vi "VNARP PARABOLA FIT.vi"(0 "Freq Table IN":dbl[](array[numeric]), 1 "Fit length":i32=500, 2 "Y IN":dbl[](array[numeric]) caption="Y") -> (3 "Best Polynomial Fit":dbl[](array[numeric]) caption="Meilleur ajustement polynomial", 4 "Parabol max position":dbl, 5 "élément":dbl, 6 "sous-tableau":dbl[](array[numeric]))   [LabVIEW 2021]
uses:
  <vilib>/Analysis/6fits.llb/General Linear Fit Algorithm.ctl
  <vilib>/Analysis/NI_AALPro.lvlib
panel:
  out "error out":errorcluster caption="sortie d'erreur"
  out "error":i32 caption="erreur"
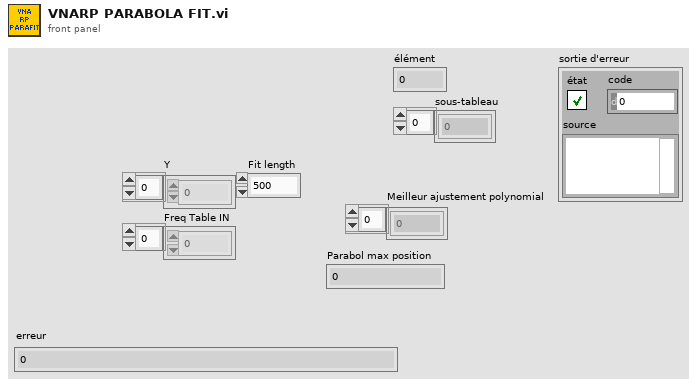
[diagram p1: front panel]
types:
  T1 = typedef "NI_AALPro.lvlib/General Linear Fit Algorithm.ctl" = u16
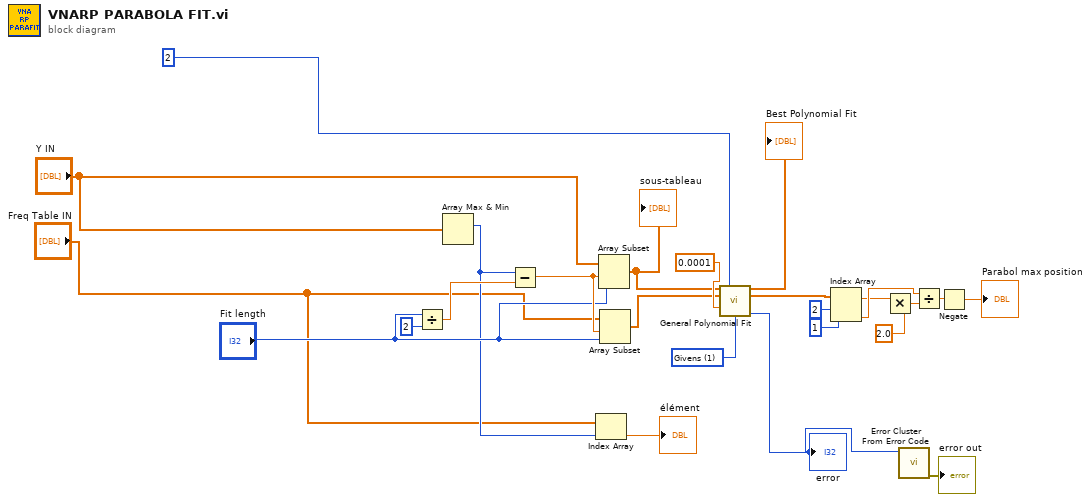
[diagram p0: block diagram]
diagram:
  w8 = T1 1 items=["SVD", "Givens", "Givens2", "Householder", "Décomposition LU", "Cholesky", "SVD pour H pas de plein rang"] ("algorithm")
  n1 = Divide(x="Fit length", y=2 ("polynomial order")) -> (x/y=w9:dbl)
  n2 = Array Max & Min(array="Y IN") -> (max index (indices)=w5:i32)  [unwired: 3 out]
  n3 = Subtract(x=w5, y=w9) -> (x-y=w21:dbl)
  n4 = Index Array(array="Freq Table IN", index=w5) -> (element=→"élément":dbl)
  n5 = Array Subset(array="Y IN", index=w21, length="Fit length") -> (w22:dbl[])
  "sous-tableau" <- w22
  n6 = Array Subset(array="Freq Table IN", index=w21, length="Fit length") -> (w23:dbl[])
  n7 = call <vilib>:"General Polynomial Fit.vi"("Y"=w22, "polynomial order"=2, "X"=w23, "tolerance"=0.0001, "algorithm"=w8) -> ("Best Polynomial Fit"=→"Best Polynomial Fit":dbl[], "Polynomial Coefficients"=w12:dbl[], "error"=w2:i32)  [unwired: 7 in, 1 out]
  "error" <- w2
  n8 = Index Array(array=w12, index #1=2 ("indice"), index #2=1 ("indice")) -> (element #1=w16:dbl, element #2=w18:dbl)
  n9 = Multiply(x=w16, y=2.0) -> (x*y=w15:dbl)
  n10 = call <vilib>:"Error Cluster From Error Code.vi"("error code (0)"=w2) -> ("error out"=→"error out":errorcluster)  [unwired: 8 in]
  n11 = Divide(x=w18, y=w15) -> (x/y=w19:dbl)
  n12 = Negate(x=w19) -> (-x=→"Parabol max position":dbl)
